vi "LaserACCcurrent.vi"(4 "ACC":dbl(slide) min=0.0 max=90.0 scale=0.0..90.0, 5 "COM Port":refnum<visa-resource-name>="COM6") -> ()   [LabVIEW 2020]
uses:
  <vilib>/Instr/_visa.llb/VISA Configure Serial Port (Instr).vi
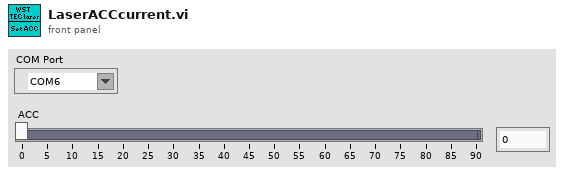
[diagram p1: front panel]
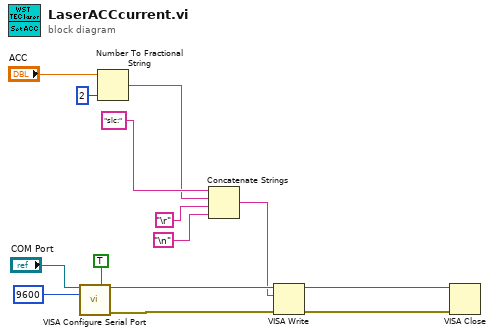
[diagram p0: block diagram]
diagram:
  n1 = call-poly "VISA Configure Serial Port"("VISA resource name"="COM Port", "Enable Termination\nChar (T)"=TRUE ("Enable Termination\nChar (T)"), "baud rate (9600)"=u32 9600) -> ("VISA resource name out"=w11:refnum<visa-resource-name>, "error out"=w10:errorcluster)  [unwired: 11 in]
  n2 = Number To Fractional String(number="ACC", precision (6)=i16 2) -> (F-format string=w1:string)  [unwired: 2 in]
  n3 = Concatenate Strings("slc:", w1, "\r", "\n") -> (w5:string)
  n4 = VISA Write(VISA resource name=w11, write buffer=w5, error in (no error)=w10) -> (VISA resource name out=w9:refnum<visa-resource-name>, error out=w8:errorcluster)  [unwired: 1 out]
  n5 = VISA Close(VISA resource name=w9, error in (no error)=w8) -> ()  [unwired: 1 out]
